vi "Match String with Wildcard Pattern List.vi"(3 "case matching (sensitive)":T1=enum."system", 4 "string":string, 5 "pattern list":string[](array[string])=["lybraryn.llb/*", "memmon.llb/*"]) -> (0 "found substring":bool, 1 "match pattern":string, 2 "index":i32)   [LabVIEW 2012, in "Car Wash.lvlib" / "Tools_String.lvlib"]
uses:
  Tools_String.lvlib
  <vilib>/FTP/util/Case Matching.ctl
  Get Case Insensitive Search Pattern.vi
  Get Wildcard Search Pattern.vi
  <vilib>/FTP/NI_FTP.lvlib
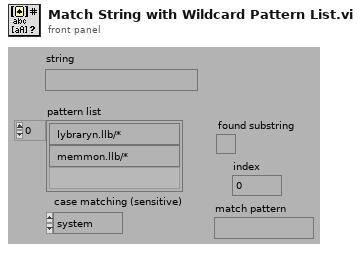
[diagram p1: front panel]
types:
  T1 = typedef "NI_FTP.lvlib/Case Matching.ctl" = enum16{"a != A", "a == A", "system"}
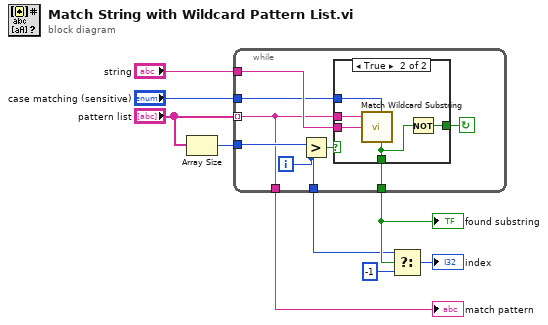
[diagram p0: block diagram]
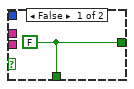
[diagram p2: hidden frame]
diagram:
  n1 = Array Size(array="pattern list") -> (size(s)=w7:i32)
  n2 = while {
    tunnel: [w11] -> w2
    tunnel: [w12] -> w4
    tunnel: [w14] -> w6
    tunnel: "string" -> [w16]
    tunnel: w7 -> [w17]
    tunnel: "pattern list" -> [w11] mode=indexing
    tunnel: "case matching (sensitive)" -> [w10]
    i -> [w12]
    stop <- w13 continue-if-true
    n3 = Greater?(x=w17, y=w12) -> (0:w15:bool)
    n4 = case shown="True" w15 {
      tunnel: w16 -> [_ w23]
      tunnel: w11 -> [_ w22]
      tunnel: [w18 w21] -> w14
      tunnel: [w18 w20] -> w13
      tunnel: w10 -> [_ w19]
      frame False {
        w18 = FALSE
      }
      frame True {
        n5 = call "Match Wildcard Substring.vi"("case matching (sensitive)"=w19, "string"=w23, "pattern with wildcards"=w22) -> ("found substring"=w21:bool)  [unwired: 1 in, 4 out]
        n6 = Not(x=w21) -> (.not. x?=w20:bool)
      }
    }
  }
  "found substring" <- w6
  "match pattern" <- w2
  n7 = Select(t=w4, s=w6, f=-1) -> (s? t:f=→"index":i32)
